vi "InitialValues.vi"(6 "Ref?":bool, 8 "error in (no error)":errorcluster, 10 "Plik?":bool, 11 "References":T1) -> (0 "error out":errorcluster)   [LabVIEW 2021]
uses:
  Typedefs/Referencias.ctl
  Typedefs/Axis.ctl
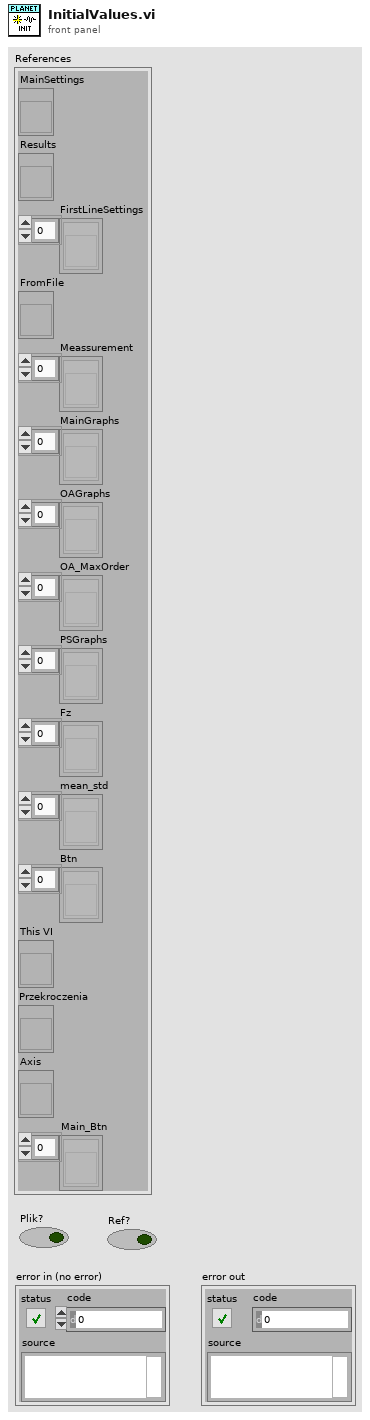
[diagram p1: front panel]
types:
  T1 = typedef "Referencias.ctl" = cluster{"MainSettings":refnum<vi>, "Results":refnum<vi>, "FirstLineSettings":refnum<vi>[], "FromFile":refnum<vi>, "Meassurement":refnum<vi>[], "MainGraphs":refnum<vi>[], "OAGraphs":refnum<vi>[], "OA_MaxOrder":refnum<vi>[], "PSGraphs":refnum<vi>[], "Fz":refnum<vi>[], "mean_std":refnum<vi>[], "Btn":refnum<vi>[], "This VI":refnum<vi>, "Przekroczenia":refnum<vi>, "Axis":refnum<vi>, "Main_Btn":refnum<vi>[]}
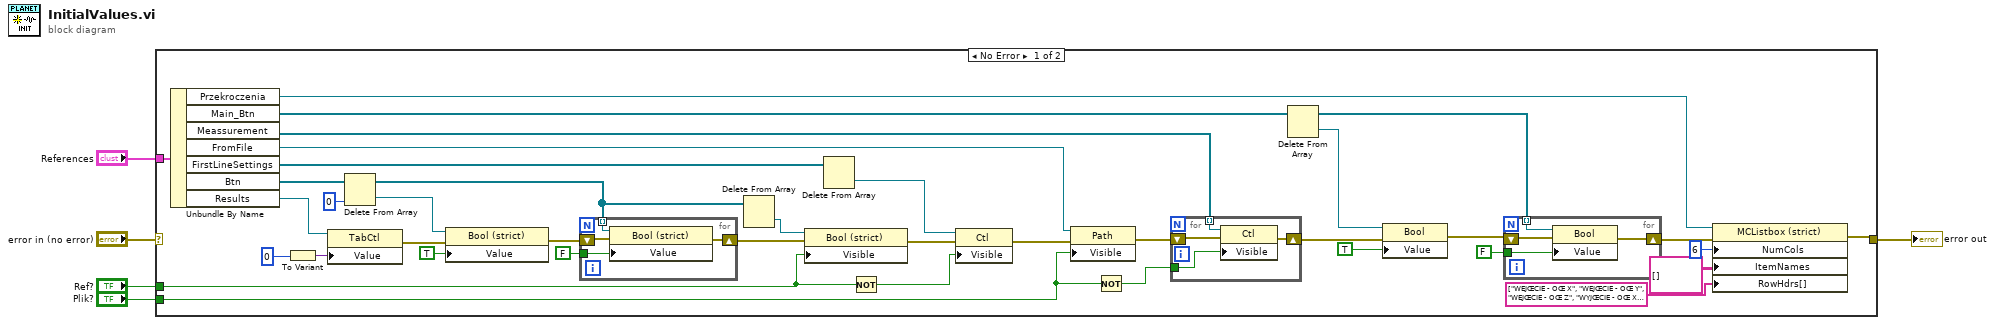
[diagram p0: block diagram]
diagram:
  n1 = case shown="No Error" "error in (no error)" {
    selector: "error in (no error)" -> [_ w56]
    tunnel: "Plik?" -> [w43 _]
    tunnel: "References" -> [w41 _]
    tunnel: [w10 w56] -> w2
    tunnel: "Ref?" -> [w13 _]
    frame No Error {
      n2 = Unbundle By Name(w41) -> ("Przekroczenia"=w9:refnum<vi>, "Main_Btn"=w32:refnum<vi>[], "Meassurement"=w42:refnum<vi>[], "FromFile"=w26:refnum<vi>, "FirstLineSettings"=w17:refnum<vi>[], "Btn"=w23:refnum<vi>[], "Results"=w37:refnum<vi>)
      n3 = To Variant(anything=0) -> (Variant=w34:variant)
      n4 = property class="TabCtl"(reference=w37, "Value"=w34) -> (error out=w36:errorcluster)  [unwired: 1 in, 1 out]
      n5 = Delete From Array(array=w23, index=0) -> (deleted portion=w22:refnum<vi>, array with subset deleted=w19:refnum<vi>[])  [unwired: 1 in]
      n6 = property class="Bool (strict)"(reference=w22, error in=w36, "Value"=TRUE) -> (error out=w25:errorcluster)  [unwired: 1 out]
      n7 = for {
        tunnel: w19 -> [w46] mode=indexing
        shift-right: [w45] -> w20
        shift-left: w25 -> [w47]
        tunnel: FALSE -> [w44]
        n8 = property class="Bool (strict)"(reference=w46, error in=w47, "Value"=w44) -> (error out=w45:errorcluster)  [unwired: 1 out]
      }
      n9 = Delete From Array(array=w19) -> (deleted portion=w18:refnum<vi>)  [unwired: 2 in, 1 out]
      n10 = property class="Bool (strict)"(reference=w18, error in=w20, "Visible"=w13) -> (error out=w15:errorcluster)  [unwired: 1 out]
      n11 = Delete From Array(array=w17) -> (deleted portion=w16:refnum<vi>)  [unwired: 2 in, 1 out]
      n12 = Not(x=w13) -> (.not. x?=w12:bool)
      n13 = property class="Ctl"(reference=w16, error in=w15, "Visible"=w12) -> (error out=w14:errorcluster)  [unwired: 1 out]
      n14 = property class="Path"(reference=w26, error in=w14, "Visible"=w43) -> (error out=w39:errorcluster)  [unwired: 1 out]
      n15 = Not(x=w43) -> (.not. x?=w40:bool)
      n16 = for {
        tunnel: w42 -> [w54] mode=indexing
        shift-right: [w53] -> w30
        shift-left: w39 -> [w55]
        tunnel: w40 -> [w52]
        n17 = property class="Ctl"(reference=w54, error in=w55, "Visible"=w52) -> (error out=w53:errorcluster)  [unwired: 1 out]
      }
      n18 = Delete From Array(array=w32) -> (deleted portion=w29:refnum<vi>, array with subset deleted=w31:refnum<vi>[])  [unwired: 2 in]
      n19 = property class="Bool"(reference=w29, error in=w30, "Value"=TRUE) -> (error out=w28:errorcluster)  [unwired: 1 out]
      n20 = for {
        tunnel: w31 -> [w50] mode=indexing
        shift-right: [w49] -> w11
        shift-left: w28 -> [w51]
        tunnel: FALSE -> [w48]
        n21 = property class="Bool"(reference=w50, error in=w51, "Value"=w48) -> (error out=w49:errorcluster)  [unwired: 1 out]
      }
      n22 = property class="MCListbox (strict)"(reference=w9, error in=w11, "NumCols"=u32 6 ("Number of Columns"), "ItemNames"=string[][] [] ("Item Names"), "RowHdrs[]"=string[] ["WEJŒCIE - OŒ X", "WEJŒCIE - OŒ Y", "WEJŒCIE - OŒ Z", "WYJŒCIE - OŒ X", "WYJŒCIE - OŒ Y", "WYJŒCIE - OŒ Z"]) -> (error out=w10:errorcluster)  [unwired: 1 out]
    }
    frame Error {
    }
  }
  "error out" <- w2
